vi "Get Device Configuration--SubVI.vi"(8 "error in (no error)":errorcluster, 10 "Device State in":T1 {"Control State"."Control Mode" items=["Bus/RS232"=0, "FLOW-BUS slave"=2, "Valve close"=3, "Controller idle"=4, "Setpoint 100%"=7, "Valve fully open"=8, "Calibration mode"=9, "Setpoint 0%"=12, "RS232"=18, "Valve steering"=20, "Valve safe state"=22]}, 11 "MB_Master_TCP in":refnum<class "MB_Master_TCP.lvclass">) -> (0 "error out":errorcluster, 2 "Device State out":T1 {"Control State"."Control Mode" items=["Bus/RS232"=0, "FLOW-BUS slave"=2, "Valve close"=3, "Controller idle"=4, "Setpoint 100%"=7, "Valve fully open"=8, "Calibration mode"=9, "Setpoint 0%"=12, "RS232"=18, "Valve steering"=20, "Valve safe state"=22]}, 3 "MB_Master_TCP out":refnum<class "MB_Master_TCP.lvclass">)   [LabVIEW 2024, in "FlexiFlowInterfaceCH2.lvlib"]
uses:
  FlexiFlowInterfaceCH2.lvlib
  Modbus Flexi-Flow State--cluster.ctl
  <vilib>/Plasmionique/MB Master/MB_Master_TCP/MB_Master_TCP.lvclass
  Device Type--enum.ctl
  Modbus Flexi-Flow Controls--cluster.ctl
  Modbus Flexi-Flow API/Control Mode--enum.ctl
  Modbus Flexi-Flow API/Control Function Values--enum.ctl
  Modbus Flexi-Flow Measure State--cluster.ctl
  Modbus Flexi-Flow API/PDU Address Char 8-bit Params--ring.ctl
  Modbus Flexi-Flow API/PDU Address U16 Params--ring.ctl
  Modbus Flexi-Flow API/PDU Address Float 32-bit Params--ring.ctl
  Modbus Flexi-Flow API/PDU Address String Params--ring.ctl
  Modbus Flexi-Flow API/Read Char Register.vi
  Modbus Flexi-Flow API/Read Unsigned Int Register.vi
  Modbus Flexi-Flow API/Read Float Register.vi
  Modbus Flexi-Flow API/Read String Register.vi
  Modbus Flexi-Flow API/Bronkhorst Flexi-Flow ModbusTCP API.lvlib
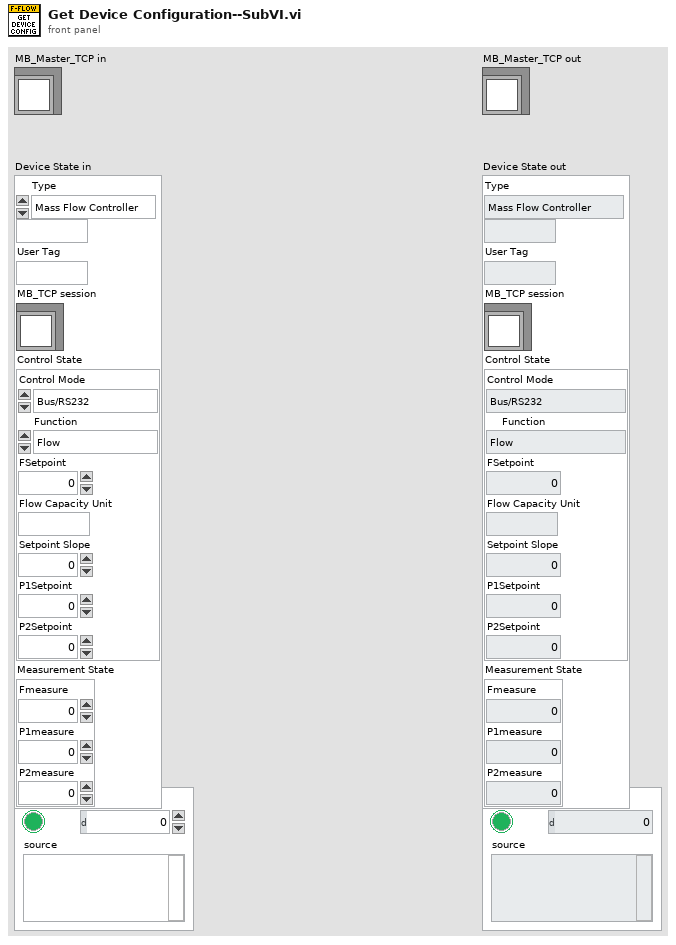
[diagram p1: front panel]
types:
  T1 = typedef "FlexiFlowInterfaceCH2.lvlib/Modbus Flexi-Flow State--cluster.ctl" = cluster{"Type":T2, "Label":string, "User Tag":string, "MB_TCP session":refnum<class "MB_Master_TCP.lvclass">, "Control State":T3, "Measurement State":T6}
  T2 = typedef "FlexiFlowInterfaceCH2.lvlib/Device Type--enum.ctl" = enum16{"Mass Flow Controller", "Mass Flow Meter"}
  T3 = typedef "FlexiFlowInterfaceCH2.lvlib/Modbus Flexi-Flow Controls--cluster.ctl" = cluster{"Control Mode":T4, "Function":T5, "FSetpoint":sgl, "Flow Capacity Unit":string, "Setpoint Slope":u16, "P1Setpoint":sgl, "P2Setpoint":sgl}
  T4 = typedef "Bronkhorst Flexi-Flow ModbusTCP API.lvlib/Control Mode--enum.ctl" = u16
  T5 = typedef "Bronkhorst Flexi-Flow ModbusTCP API.lvlib/Control Function Values--enum.ctl" = enum16{"Flow", "Upstream pressure", "Downstream pressure", "Flow with upstream pressure limit", "Flow with downstream pressure limit", "Upstream pressure with flow limit", "Downstream pressure with flow limit"}
  T6 = typedef "FlexiFlowInterfaceCH2.lvlib/Modbus Flexi-Flow Measure State--cluster.ctl" = cluster{"Fmeasure":dbl, "P1measure":sgl, "P2measure":sgl}
  T7 = typedef "Bronkhorst Flexi-Flow ModbusTCP API.lvlib/Fmeasure (F,P1,P2)--cluster.ctl" = cluster{"Fmeasure (F)":sgl, "Fmeasure (P1)":sgl, "Fmeasure (P2)":sgl}
  T8 = typedef "Bronkhorst Flexi-Flow ModbusTCP API.lvlib/PDU Address Char 8-bit Params--ring.ctl" = u16
  T9 = typedef "Bronkhorst Flexi-Flow ModbusTCP API.lvlib/PDU Address U16 Params--ring.ctl" = u16
  T10 = typedef "Bronkhorst Flexi-Flow ModbusTCP API.lvlib/PDU Address Float 32-bit Params--ring.ctl" = u16
  T11 = typedef "Bronkhorst Flexi-Flow ModbusTCP API.lvlib/PDU Address String Params--ring.ctl" = u16
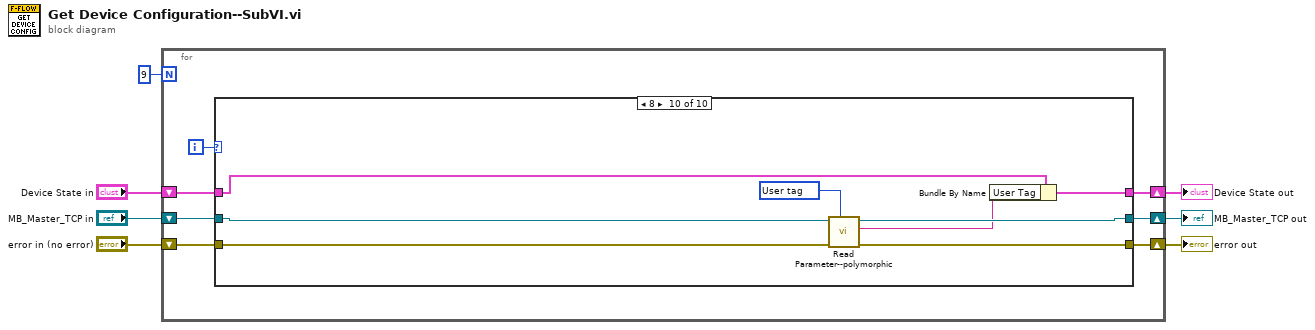
[diagram p0: block diagram]
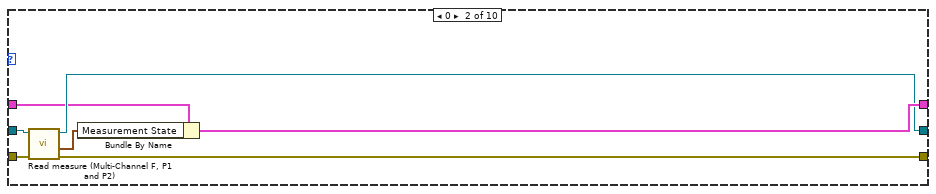
[diagram p3: hidden frame]
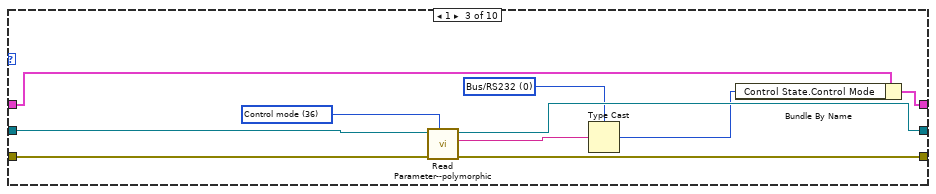
[diagram p4: hidden frame]
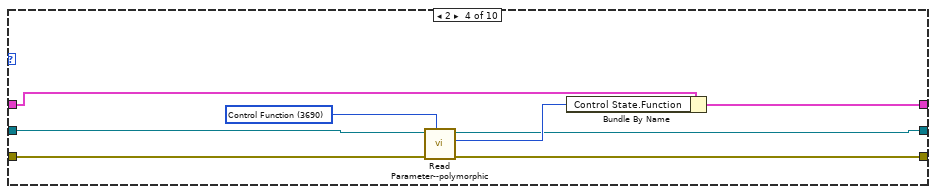
[diagram p5: hidden frame]
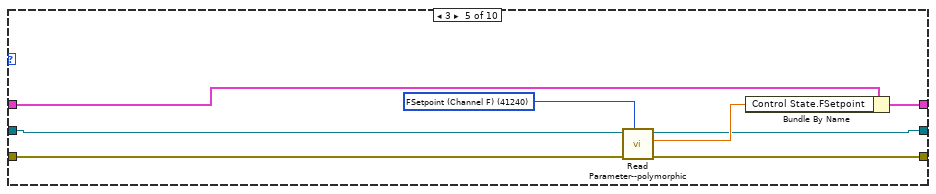
[diagram p6: hidden frame]
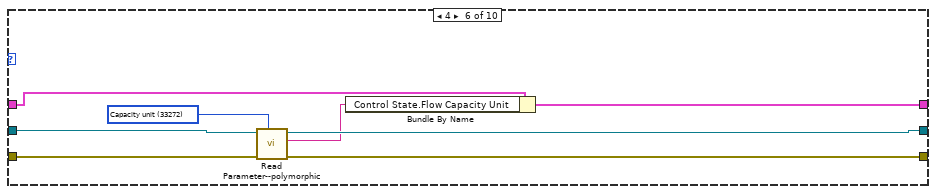
[diagram p7: hidden frame]
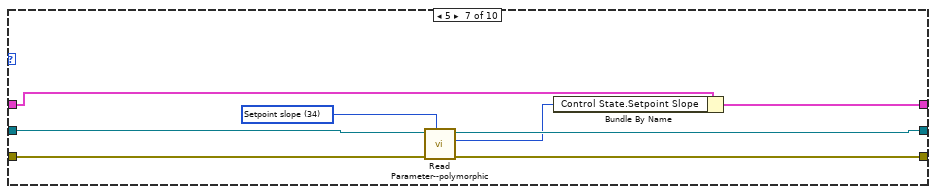
[diagram p8: hidden frame]
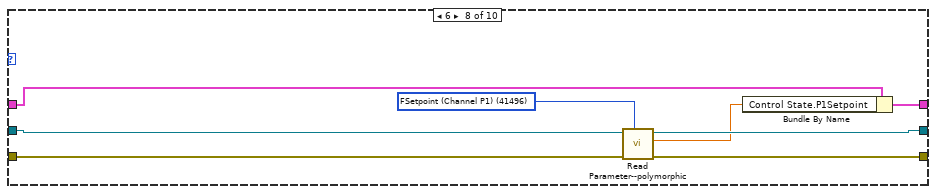
[diagram p9: hidden frame]
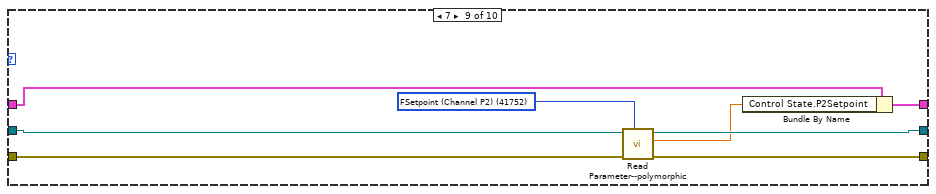
[diagram p10: hidden frame]
diagram:
  n1 = for {
    N: 9 -> [_]
    shift-right: [w14] -> w7
    shift-left: "error in (no error)" -> [w13]
    shift-right: [w11] -> w4
    shift-left: "MB_Master_TCP in" -> [w10]
    shift-right: [w12] -> w5
    shift-left: "Device State in" -> [w9]
    i -> [w8]
    n2 = case shown="8" w8 {
      tunnel: [w15 w24 w30 w35 w46 w53 w62 w70 w78 w86] -> w14
      tunnel: w13 -> [w15 w23 w31 w36 w47 w52 w61 w69 w77 w85]
      tunnel: [w17 w22 w28 w41 w49 w57 w65 w73 w81 w89] -> w12
      tunnel: [w16 w20 w32 w38 w44 w54 w63 w71 w79 w87] -> w11
      tunnel: w10 -> [w16 w19 w33 w37 w43 w55 w64 w72 w80 w88]
      tunnel: w9 -> [w17 w18 w29 w42 w50 w58 w66 w74 w82 w90]
      frame Default {
      }
      frame 0 {
        n3 = call "Read measure (Multi-Channel F, P1 and P2).vi"("error in"=w23, "MB_TCP session in"=w19) -> ("error out"=w24:errorcluster, "Fmeasure (F, P1, P2)"=w21:T7, "MB session out"=w20:refnum<class "MB_Master_TCP.lvclass">)  [unwired: 7 in]
        n4 = Bundle By Name(cluster=w18, "Measurement State"=w21) -> (w22:T1)
      }
      frame 1 {
        w26 = T4 0 items=["Bus/RS232"=0, "FLOW-BUS slave"=2, "Valve close"=3, "Controller idle"=4, "Setpoint 100%"=7, "Valve fully open"=8, "Calibration mode"=9, "Setpoint 0%"=12, "RS232"=18, "Valve steering"=20, "Valve safe state"=22] ("Control State.Control Mode")
        w34 = T8 36 items=["Wink"=0, "Control mode"=36, "Alarm mode"=3107, "Alarm setpoint"=3109, "Reset alarm enable"=3113, "Counter unit index"=3330, "Counter setpoint mode"=3333, "Counter mode"=3336, "Reset counter enable"=3337, "Reset"=3688, "Modbus slave address"=4010] ("PDU Address Char 8-bit")
        n5 = call-poly "Read Parameter--polymorphic.vi"("PDU Address Char 8-bit"=w34, "error in"=w31, "MB_TCP session in"=w33) -> ("error out"=w30:errorcluster, "Unsigned Char"=w27:string, "MB session out"=w32:refnum<class "MB_Master_TCP.lvclass">)  [unwired: 6 in]
        n6 = Type Cast(type=w26, x=w27) -> (*(type *) &x=w25:T4)
        n7 = Bundle By Name(cluster=w29, "Control State.Control Mode"=w25) -> (w28:T1)
      }
      frame 2 {
        w40 = T9 3690 items=["Setpoint"=33, "Setpoint slope"=34, "Alarm limit maximum"=3105, "Alarm limit minimum"=3106, "Alarm new setpoint"=3110, "Counter limit (UInt)"=3331, "Counter new setpoint"=3334, "Valve output"=61960, "Control Function"=3690, "TEMP"=0] ("PDU Address (U-Int16)")
        n8 = call-poly "Read Parameter--polymorphic.vi"("PDU Address (U-Int16)"=w40, "error in"=w36, "MB_TCP session in"=w37) -> ("error out"=w35:errorcluster, "Value"=w39:u16, "MB session out"=w38:refnum<class "MB_Master_TCP.lvclass">)  [unwired: 6 in]
        n9 = Bundle By Name(cluster=w42, "Control State.Function"=w39) -> (w41:T1)
      }
      frame 3 {
        w48 = T10 41240 items=["Counter New Setpoint"=3334, "FSetpoint (Channel F)"=41240, "Fmeasure (Channel F)"=41216, "FSetpoint (Channel P1)"=41496, "Fmeasure (Channel P1)"=41472, "FSetpoint (Channel P2)"=41752, "Fmeasure (Channel P2)"=41728, "Capacity 0%"=41392, "Counter value (Float)"=59400, "Counter limit (Float)"=59416, "Inlet Pressure"=61801, "Outlet Pressure"=61809, "PID-Kp"=62120, "PID-Ti"=62128, "PID-Td"=62136, "Dynamic display factor"=62728, "Static display factor"=62736, "Exponential smoothing"=62752] ("PDU Address 32-bit Float")
        n10 = call-poly "Read Parameter--polymorphic.vi"("PDU Address 32-bit Float"=w48, "error in"=w47, "MB_TCP session in"=w43) -> ("error out"=w46:errorcluster, "Value"=w45:sgl, "MB session out"=w44:refnum<class "MB_Master_TCP.lvclass">)  [unwired: 6 in]
        n11 = Bundle By Name(cluster=w50, "Control State.FSetpoint"=w45) -> (w49:T1)
      }
      frame 4 {
        w56 = T11 33272 items=["Fluid name"=33160, "Capacity unit"=33272, "Counter unit"=59448, "User tag"=61744] ("PDU Address String Params")
        n12 = call-poly "Read Parameter--polymorphic.vi"("PDU Address String Params"=w56, "error in"=w52, "MB_TCP session in"=w55) -> ("error out"=w53:errorcluster, "Value"=w51:string, "MB session out"=w54:refnum<class "MB_Master_TCP.lvclass">)  [unwired: 6 in]
        n13 = Bundle By Name(cluster=w58, "Control State.Flow Capacity Unit"=w51) -> (w57:T1)
      }
      frame 5 {
        w60 = T9 34 items=["Setpoint"=33, "Setpoint slope"=34, "Alarm limit maximum"=3105, "Alarm limit minimum"=3106, "Alarm new setpoint"=3110, "Counter limit (UInt)"=3331, "Counter new setpoint"=3334, "Valve output"=61960, "Control Function"=3690, "TEMP"=0] ("PDU Address (U-Int16)")
        n14 = call-poly "Read Parameter--polymorphic.vi"("PDU Address (U-Int16)"=w60, "error in"=w61, "MB_TCP session in"=w64) -> ("error out"=w62:errorcluster, "Value"=w59:u16, "MB session out"=w63:refnum<class "MB_Master_TCP.lvclass">)  [unwired: 6 in]
        n15 = Bundle By Name(cluster=w66, "Control State.Setpoint Slope"=w59) -> (w65:T1)
      }
      frame 6 {
        w67 = T10 41496 items=["Counter New Setpoint"=3334, "FSetpoint (Channel F)"=41240, "Fmeasure (Channel F)"=41216, "FSetpoint (Channel P1)"=41496, "Fmeasure (Channel P1)"=41472, "FSetpoint (Channel P2)"=41752, "Fmeasure (Channel P2)"=41728, "Capacity 0%"=41392, "Counter value (Float)"=59400, "Counter limit (Float)"=59416, "Inlet Pressure"=61801, "Outlet Pressure"=61809, "PID-Kp"=62120, "PID-Ti"=62128, "PID-Td"=62136, "Dynamic display factor"=62728, "Static display factor"=62736, "Exponential smoothing"=62752] ("PDU Address 32-bit Float")
        n16 = call-poly "Read Parameter--polymorphic.vi"("PDU Address 32-bit Float"=w67, "error in"=w69, "MB_TCP session in"=w72) -> ("error out"=w70:errorcluster, "Value"=w68:sgl, "MB session out"=w71:refnum<class "MB_Master_TCP.lvclass">)  [unwired: 6 in]
        n17 = Bundle By Name(cluster=w74, "Control State.P1Setpoint"=w68) -> (w73:T1)
      }
      frame 7 {
        w75 = T10 41752 items=["Counter New Setpoint"=3334, "FSetpoint (Channel F)"=41240, "Fmeasure (Channel F)"=41216, "FSetpoint (Channel P1)"=41496, "Fmeasure (Channel P1)"=41472, "FSetpoint (Channel P2)"=41752, "Fmeasure (Channel P2)"=41728, "Capacity 0%"=41392, "Counter value (Float)"=59400, "Counter limit (Float)"=59416, "Inlet Pressure"=61801, "Outlet Pressure"=61809, "PID-Kp"=62120, "PID-Ti"=62128, "PID-Td"=62136, "Dynamic display factor"=62728, "Static display factor"=62736, "Exponential smoothing"=62752] ("PDU Address 32-bit Float")
        n18 = call-poly "Read Parameter--polymorphic.vi"("PDU Address 32-bit Float"=w75, "error in"=w77, "MB_TCP session in"=w80) -> ("error out"=w78:errorcluster, "Value"=w76:sgl, "MB session out"=w79:refnum<class "MB_Master_TCP.lvclass">)  [unwired: 6 in]
        n19 = Bundle By Name(cluster=w82, "Control State.P2Setpoint"=w76) -> (w81:T1)
      }
      frame 8 {
        w83 = T11 61744 items=["Fluid name"=33160, "Capacity unit"=33272, "Counter unit"=59448, "User tag"=61744] ("PDU Address String Params")
        n20 = call-poly "Read Parameter--polymorphic.vi"("PDU Address String Params"=w83, "error in"=w85, "MB_TCP session in"=w88) -> ("error out"=w86:errorcluster, "Value"=w84:string, "MB session out"=w87:refnum<class "MB_Master_TCP.lvclass">)  [unwired: 6 in]
        n21 = Bundle By Name(cluster=w90, "User Tag"=w84) -> (w89:T1)
      }
    }
  }
  "error out" <- w7
  "Device State out" <- w5
  "MB_Master_TCP out" <- w4
